vi "mod3 (1).vi"() -> ()   [LabVIEW 2014]
doc: "\"Discrete LED demo.vi\" -- Demonstrate a discrete LED connected to a digital output.\n\nInstructions:\n\n-- Click the 'enable blinker' button to toggle between blinking mode\nand static mode.\n-- In static mode, click the 'digital level' button to set the state of the\ndigital output.\n-- The 'digital output state' LED indicator shows the state of the\ndigital output (on = high, off = low)."
uses:
  <vilib>/myRIO/Common/Instrument Driver Framework/myRIO v1.0/UART/vis/myRIO v1.0 Close UART.vi
  <vilib>/myRIO/Common/Instrument Driver Framework/Utilities/vis/FPGA Ref Manager.vi
  <vilib>/myRIO/Common/Instrument Driver Framework/myRIO v1.0/myRIO v1.0 Reset FPGA.vi
  <vilib>/myRIO/Common/Instrument Driver Framework/myRIO v1.0/IRQ/vis/myRIO v1.0 IRQ Info FGV.vi
  <vilib>/myRIO/Common/Instrument Driver Framework/myRIO v1.0/IRQ/vis/myRIO v1.0 Timer IRQ Info FGV.vi
  <vilib>/myRIO/Common/Instrument Driver Framework/myRIO v1.0/IRQ/vis/myRIO v1.0 ISR Agent.vi
  <vilib>/Utility/error.llb/Error Cluster From Error Code.vi
  <vilib>/myRIO/Common/Instrument Driver Framework/myRIO v1.0/DIO/vis/myRIO v1.0 Write DIO.vi
  <vilib>/myRIO/Instrument Drivers/Utilities/Utilities.lvlib
  <vilib>/myRIO/Instrument Drivers/Onboard IO/DIO/DIO.lvlib
panel:
  in  "Numeric  0,-9":u16
  out "error out":errorcluster
  in  "error in (no error)":errorcluster
  in  "[ESC]":bool
  # "7-Segment LED demo"
  # "segment 'a'"
  # "segment 'b'"
  # "segment 'c'"
  # "segment 'd'"
  # "segment 'e'"
  # "segment 'f'"
  # "segment 'g'"
  # "decimal point"
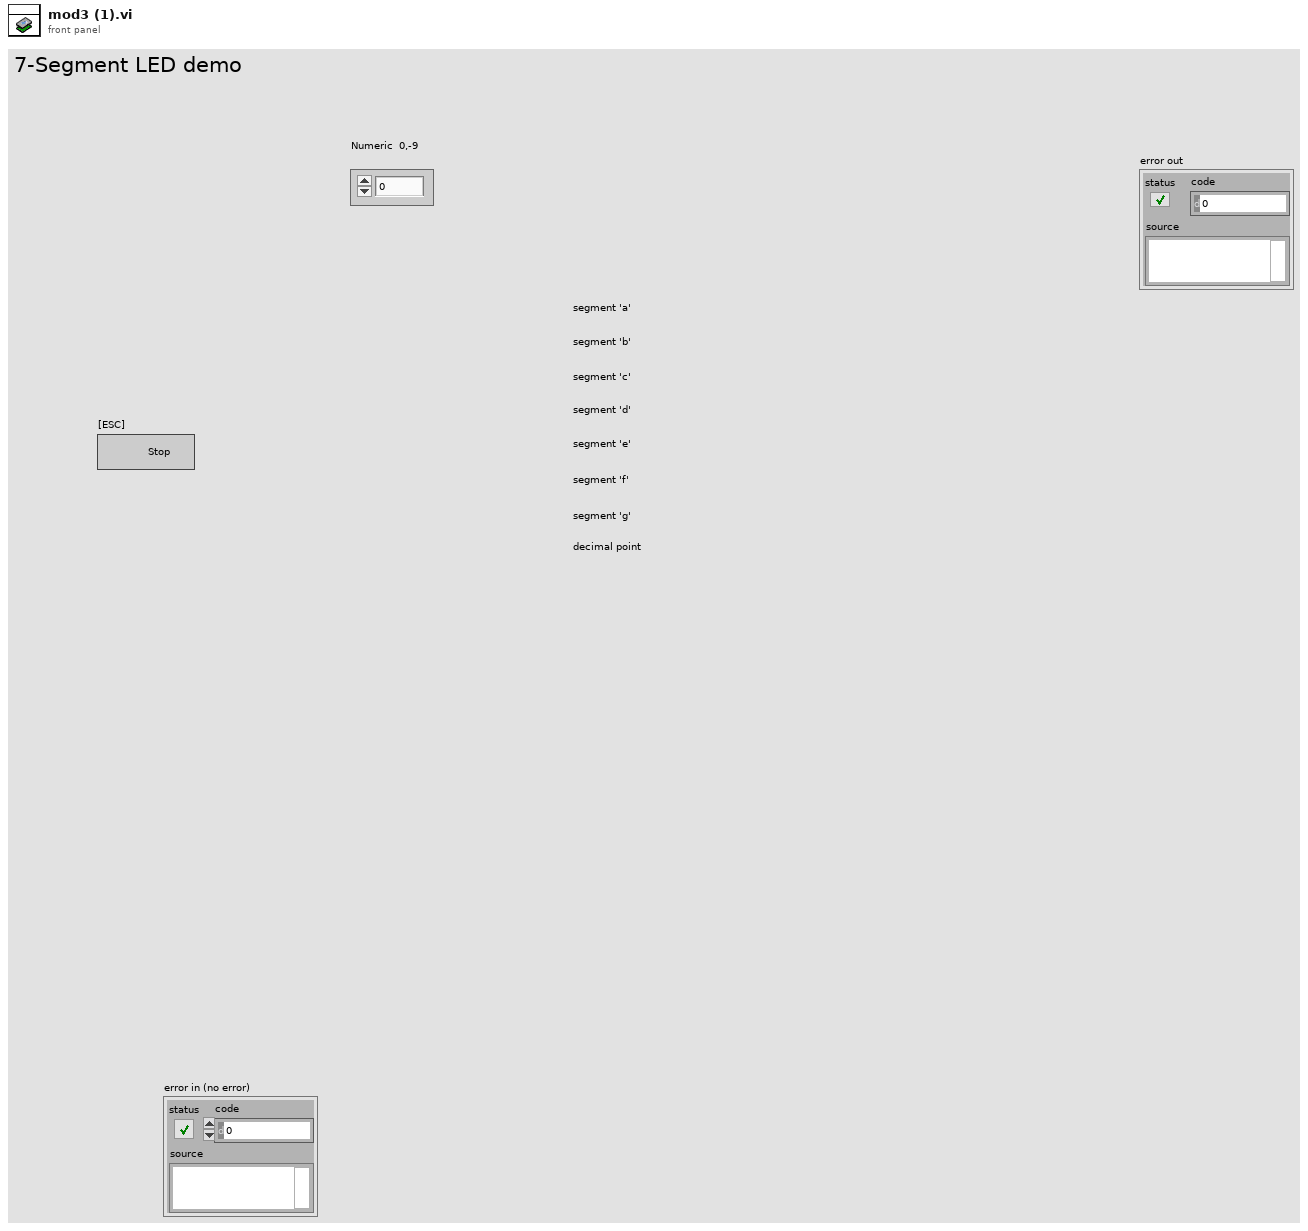
[diagram p1: front panel]
types:
  T1 = typedef "DIO.lvlib/DIO Reference.ctl" = cluster{"myRIO Reference":T2, "DIO Channels List":T6}
  T2 = typedef "myRIO Generic Hardware Reference.ctl" = cluster{"myRIO Model":T3, "myRIO Hardware Reference":T4}
  T3 = typedef "Hardware Version Enum.ctl" = enum16{"Unknown", "myRIO-1900", "myRIO-1950"}
  T4 = typedef "myRIO v1.0 Reference.ctl" = cluster{"Generic FPGA Reference":T5, "Allow multiple opens":bool}
  T5 = typedef "Generic FPGA Reference.ctl" = refnum<k20>
  T6 = typedef "DIO Channels List.ctl" = T7[]
  T7 = typedef "DIO Channels Enum.ctl" = enum16{"Not Connected", "C/DIO0", "C/DIO1", "C/DIO2", "C/DIO3", "C/DIO4", "C/DIO5", "C/DIO6", "C/DIO7", "A/DIO0", "A/DIO1", "A/DIO2", "A/DIO3", "A/DIO4", "A/DIO5", "A/DIO6", "A/DIO7", "A/DIO8", "A/DIO9", "A/DIO10", "A/DIO11", "A/DIO12", "A/DIO13", "A/DIO14", "A/DIO15", "B/DIO0", "B/DIO1", "B/DIO2", "B/DIO3", "B/DIO4", "B/DIO5", "B/DIO6", "B/DIO7", "B/DIO8", "B/DIO9", "B/DIO10", "B/DIO11", "B/DIO12", "B/DIO13", "B/DIO14", "B/DIO15", "LED0", "LED1", "LED2", "LED3", "Button0"}
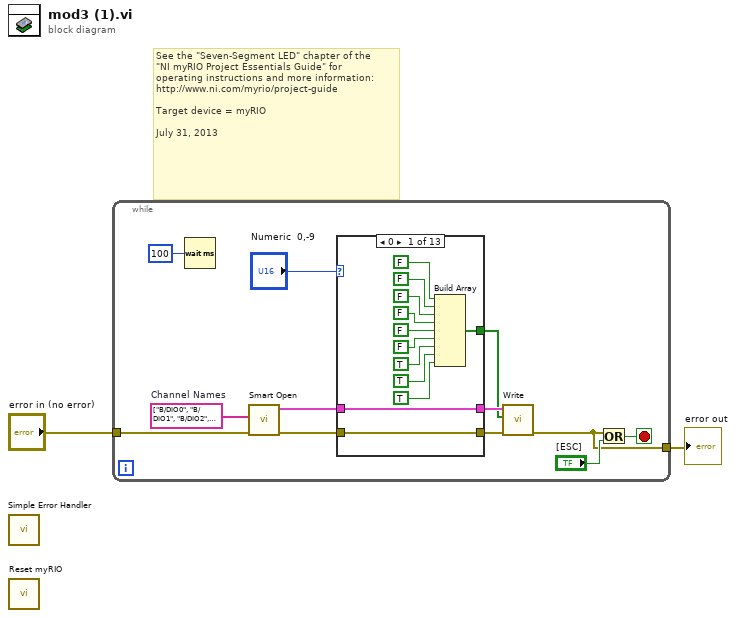
[diagram p0: block diagram]
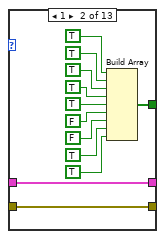
[diagram p2: hidden frame]
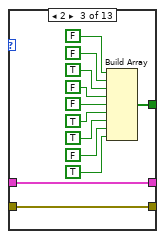
[diagram p3: hidden frame]
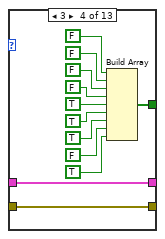
[diagram p4: hidden frame]
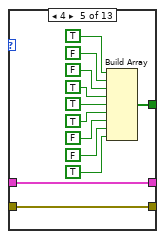
[diagram p5: hidden frame]
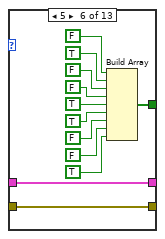
[diagram p6: hidden frame]
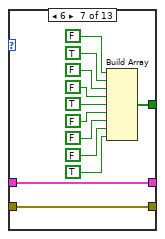
[diagram p7: hidden frame]
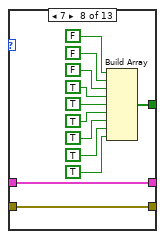
[diagram p8: hidden frame]
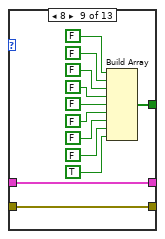
[diagram p9: hidden frame]
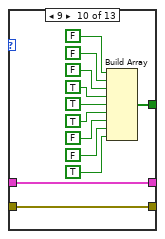
[diagram p10: hidden frame]
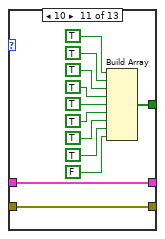
[diagram p11: hidden frame]
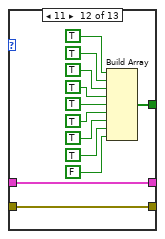
[diagram p12: hidden frame]
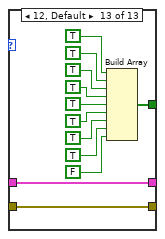
[diagram p13: hidden frame]
diagram:
  # "See the \"Seven-Segment LED\" chapter of the\n\"NI myRIO Project Essentials Guide\" for\noperating instructions and more information: \nhttp://www.ni.com/myrio/project-guide\n\nTarget device = myRIO\n\nJuly 31, 2013"
  n1 = call <vilib>:"Simple Error Handler.vi"() -> ()  [unwired: 5 in, 5 out]
  n2 = call <vilib>:"Reset myRIO.vi"() -> ()  [unwired: 11 in, 1 out]
  n3 = while {
    tunnel: [w11] -> w2
    tunnel: "error in (no error)" -> [w4]
    stop <- w14 stop-if-true
    w7 = tag[] ["B/DIO0", "B/DIO1", "B/DIO2", "B/DIO3", "B/DIO4", "B/DIO5", "B/DIO6", "B/DIO7"]  # Channel Names
    n4 = Wait (ms)(milliseconds to wait=u32 100) -> ()  [unwired: 1 out]
    n5 = call <vilib>:"Smart Open.vi"("error in (no error)"=w4, "Channel Names"=w7) -> ("error out"=w10:errorcluster, "DIO Ref Out"=w8:T1)  [unwired: 8 in]
    n6 = case shown="0" "Numeric  0,-9" {
      tunnel: [w25 w37 w49 w61 w73 w85 w97 w109 w121 w133 w145 w157 w169] -> w3
      tunnel: w10 -> [w15 w27 w39 w52 w63 w75 w87 w99 w111 w124 w135 w148 w159]
      tunnel: w8 -> [w16 w28 w40 w51 w64 w76 w88 w100 w112 w123 w136 w147 w160]
      tunnel: [w16 w28 w40 w51 w64 w76 w88 w100 w112 w123 w136 w147 w160] -> w6
      tunnel: [w15 w27 w39 w52 w63 w75 w87 w99 w111 w124 w135 w148 w159] -> w5
      frame 0 {
        n7 = Build Array(FALSE, FALSE, FALSE, FALSE, FALSE, FALSE, TRUE, TRUE, TRUE) -> (w25:bool[])
      }
      frame 1 {
        n8 = Build Array(TRUE, TRUE, TRUE, TRUE, TRUE, FALSE, FALSE, TRUE, TRUE) -> (w37:bool[])
      }
      frame 2 {
        n9 = Build Array(FALSE, FALSE, TRUE, FALSE, FALSE, TRUE, TRUE, FALSE, TRUE) -> (w49:bool[])
      }
      frame 3 {
        n10 = Build Array(FALSE, FALSE, FALSE, FALSE, TRUE, TRUE, TRUE, FALSE, TRUE) -> (w61:bool[])
      }
      frame 4 {
        n11 = Build Array(TRUE, FALSE, FALSE, TRUE, TRUE, TRUE, FALSE, FALSE, TRUE) -> (w73:bool[])
      }
      frame 5 {
        n12 = Build Array(FALSE, TRUE, FALSE, FALSE, TRUE, TRUE, FALSE, FALSE, TRUE) -> (w85:bool[])
      }
      frame 6 {
        n13 = Build Array(FALSE, TRUE, FALSE, FALSE, TRUE, FALSE, FALSE, FALSE, TRUE) -> (w97:bool[])
      }
      frame 7 {
        n14 = Build Array(FALSE, FALSE, FALSE, TRUE, TRUE, TRUE, TRUE, TRUE, TRUE) -> (w109:bool[])
      }
      frame 8 {
        n15 = Build Array(FALSE, FALSE, FALSE, FALSE, FALSE, FALSE, FALSE, FALSE, TRUE) -> (w121:bool[])
      }
      frame 9 {
        n16 = Build Array(FALSE, FALSE, FALSE, TRUE, TRUE, TRUE, FALSE, FALSE, TRUE) -> (w133:bool[])
      }
      frame 10 {
        n17 = Build Array(TRUE, TRUE, TRUE, TRUE, TRUE, TRUE, TRUE, TRUE, FALSE) -> (w145:bool[])
      }
      frame 11 {
        n18 = Build Array(TRUE, TRUE, TRUE, TRUE, TRUE, TRUE, TRUE, TRUE, FALSE) -> (w157:bool[])
      }
      frame 12, Default {
        n19 = Build Array(TRUE, TRUE, TRUE, TRUE, TRUE, TRUE, TRUE, TRUE, FALSE) -> (w169:bool[])
      }
    }
    n20 = call <vilib>:"Write.vi"("error in (no error)"=w5, "Values"=w3, "DIO Ref In"=w6) -> ("error out"=w11:errorcluster)  [unwired: 6 in, 1 out]
    n21 = Or(x=w11, y="[ESC]") -> (x .or. y?=w14:bool)
  }
  "error out" <- w2
